vi "Get Version.vi"() -> (0 "versionString":string)   [LabVIEW 2020, in "zstd.lvlib"]
uses:
  zstd.lvlib
  libzstd.dll
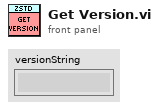
[diagram p1: front panel]
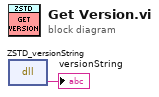
[diagram p0: block diagram]
diagram:
  n1 = dll-call lib="D:/Workspace/LabVIEW/LVToolset/vi.lib/zstd/libzstd.dll" fn="ZSTD_versionString"() -> ("return"=→"versionString":string)  [unwired: 3 in, 2 out]
